vi "002_while_loop_inside_other_btn.vi"() -> ()   [LabVIEW 2024]
panel:
  in  "Boolean":bool
  in  "stop":bool
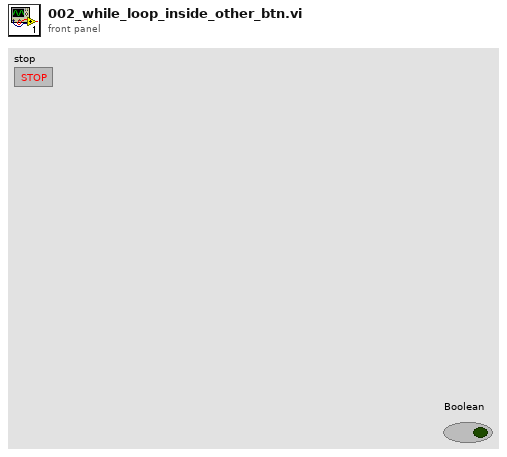
[diagram p1: front panel]
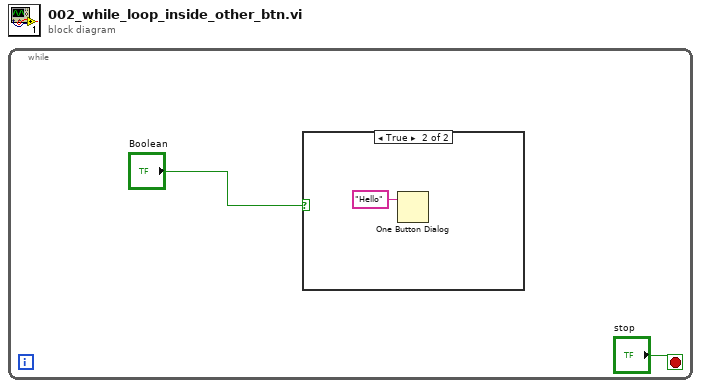
[diagram p0: block diagram]
diagram:
  n1 = while {
    stop <- "stop" stop-if-true
    n2 = case shown="True" "Boolean" {
      frame False {
      }
      frame True {
        n3 = One Button Dialog(message="Hello") -> ()  [unwired: 1 in, 1 out]
      }
    }
  }
